vi "Simple NATS Client Reader.vi"() -> ()   [LabVIEW 2018]
uses:
  <vilib>/NATS/NATS Core/Controls/nats message.ctl
  <vilib>/NATS/NATS Core/Controls/msg type.ctl
  <vilib>/NATS/NATS Core/VIs/subVIs/Set Timeout.vi
  <vilib>/NATS/NATS Core/VIs/subVIs/Validate CONNECT.vi
  <vilib>/NATS/NATS Core/VIs/NATS PING.vi
  <vilib>/dlg_ctls.llb/Space Constant.vi
  <vilib>/NATS/NATS Core/VIs/subVIs/Check for Authorization.vi
  <vilib>/NATS/NATS Core/VIs/subVIs/Add Version and Language JSON Entries.vi
  <vilib>/NATS/NATS Core/VIs/subVIs/Package Version Constant.vi
  <vilib>/Utility/error.llb/Trim Whitespace.vi
  <vilib>/NATS/NATS Core/NATS Core.lvlib
panel:
  out "nats message (MSG)":T1
  out "nats message (non-MSG)":T1
  in  "subject":string="TestSubject"
  in  "sub id":string="UniqueID-123"
  in  "timeout ms (5000)":i32=5000
  in  "port (4222)":u16=4222
  in  "NATS server address":string="localhost"
  out "error out":errorcluster
  in  "stop":bool
  # "Set prior to execution"
  # "Received messages"
  # "Visit https://nats.io to download the free, open-source NATS server"
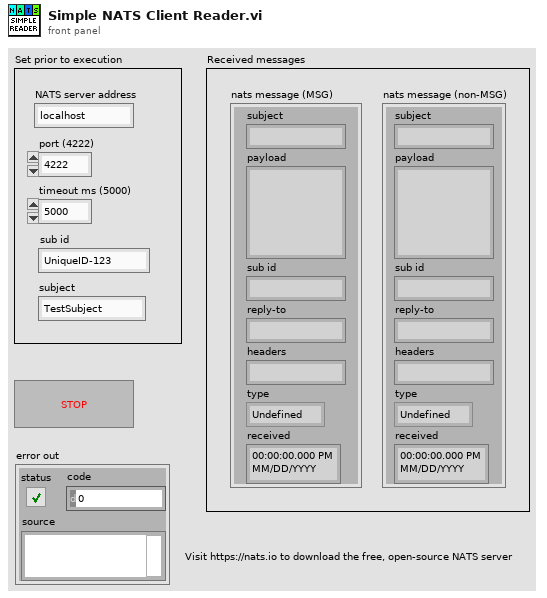
[diagram p1: front panel]
types:
  T1 = typedef "NATS Core.lvlib/nats message.ctl" = cluster{"subject":string, "payload":string, "sub id":string, "reply-to":string, "headers":string, "type":T2, "received":timestamp}
  T2 = typedef "NATS Core.lvlib/msg type.ctl" = enum16{"Undefined", "MSG", "HMSG", "+OK", "PING", "PONG", "-ERR", "INFO"}
  T3 = typedef "NATS Core.lvlib/nats connection.ctl" = cluster{"connection ID":refnum<k5>, "server INFO":string, "timeout ms":i32, "verbose?":bool, "server headers?":bool, "client headers?":bool}
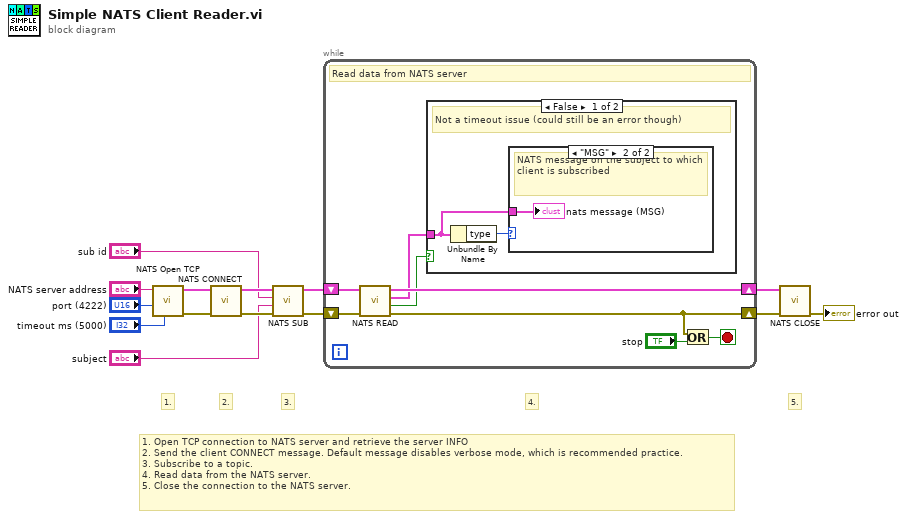
[diagram p0: block diagram]
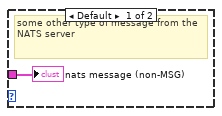
[diagram p2: hidden frame]
diagram:
  # "1. Open TCP connection to NATS server and retrieve the server INFO\n2. Send the client CONNECT message. Default message disables verbose mode, which is recommended practice.\n3. Subscribe to a topic.\n4. Read data from the NATS server.\n5. Close the connection to the NATS server."
  # "5."
  # "4."
  # "3."
  # "2."
  # "1."
  n1 = call <vilib>:"NATS Open TCP.vi"("timeout ms (5000)"="timeout ms (5000)", "port (4222)"="port (4222)", "address"="NATS server address") -> ("error out"=w11:errorcluster, "nats connection"=w14:T3)  [unwired: 5 in, 2 out]
  n2 = call <vilib>:"NATS CONNECT.vi"("error in"=w11, "nats connection in"=w14) -> ("error out"=w10:errorcluster, "nats connection out"=w13:T3)  [unwired: 7 in, 1 out]
  n3 = call <vilib>:"NATS SUB.vi"("error in"=w10, "subject"="subject", "sub id"="sub id", "nats connection in"=w13) -> ("error out"=w9:errorcluster, "dup nats connection"=w12:T3)  [unwired: 5 in, 1 out]
  n4 = while {
    shift-right: [w20] -> w8
    shift-left: w12 -> [w21]
    shift-right: [w18] -> w7
    shift-left: w9 -> [w19]
    stop <- w17 stop-if-true
    # "Read data from NATS server"
    n5 = call <vilib>:"NATS READ.vi"("error in"=w19, "nats connection in"=w21) -> ("error out"=w18:errorcluster, "timeout?"=w16:bool, "nats message"=w15:T1, "nats connection out"=w20:T3)  [unwired: 6 in]
    n6 = case shown="False" w16 {
      tunnel: w15 -> [w23 _]
      frame False {
        # "Not a timeout issue (could still be an error though)"
        n7 = Unbundle By Name(w23) -> ("type"=w24:T2)
        n8 = case shown="\"MSG\"" w24 {
          tunnel: w23 -> [w25 w26]
          frame Default {
            # "some other type of message from the NATS server"
            "nats message (non-MSG)" <- w25
          }
          frame "MSG" {
            # "NATS message on the subject to which client is subscribed"
            "nats message (MSG)" <- w26
          }
        }
      }
      frame True {
        # "Timeout -- no traffic received"
      }
    }
    n9 = Or(x=w18, y="stop") -> (x .or. y?=w17:bool)
  }
  n10 = call <vilib>:"NATS CLOSE.vi"("error in"=w7, "nats connection in"=w8) -> ("error out"=→"error out":errorcluster)  [unwired: 9 in]
